vi "Get Block Size.vi"(11 "Hash Function in":refnum<class "NI_SHA-3.lvclass">) -> (2 "block size (bytes)":i32, 3 "Hash Function out":refnum<class "NI_SHA-3.lvclass">)   [LabVIEW 2020, in "NI_SHA-3.lvclass"]
doc: "Return the hash function's input block size in bytes."
uses:
  <vilib>/security/Message Digest/SHA-3/NI_SHA-3.lvclass
  <vilib>/security/Message Digest/SHA-3/NI_SHA-3.lvclass/NI_SHA-3.ctl
  eb1e6525-3e01-40a8-a5c2-e849aaf68d04.vi
  eb1e6525-3e01-40a8-a5c2-e849aaf68d04.vi/00efce51-7697-47ef-971b-245e50795e7f.vi
  <vilib>/security/Message Digest/SHA-3/subVIs/Get Capacity.vi
  <vilib>/security/Message Digest/SHA-3/subVIs/Get Word Type.vi
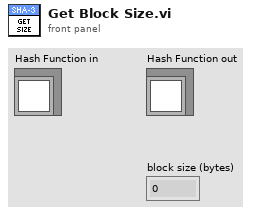
[diagram p1: front panel]
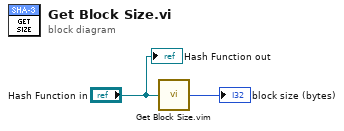
[diagram p0: block diagram]
diagram:
  n1 = call "Get Block Size.vim"("Hash Function in"="Hash Function in") -> ("block size (rate)"=→"block size (bytes)":i32)
  "Hash Function out" <- "Hash Function in"
